vi "PeriodicFilter-Check Key.vi"(7 "seconds since 1Jan1904 2":timestamp, 10 "key":string, 11 "data in":T1 {"LastCheckT" format="%<%.3X>T"}) -> (0 "index":i32, 3 "data out":T1 {"LastCheckT" format="%<%.3X>T"})   [LabVIEW 2017, in "Communicable State Machine.lvlib"]
uses:
  Communicable State Machine.lvlib
  Periodic String Filter Data.ctl
  Periodic String Filter Info.ctl
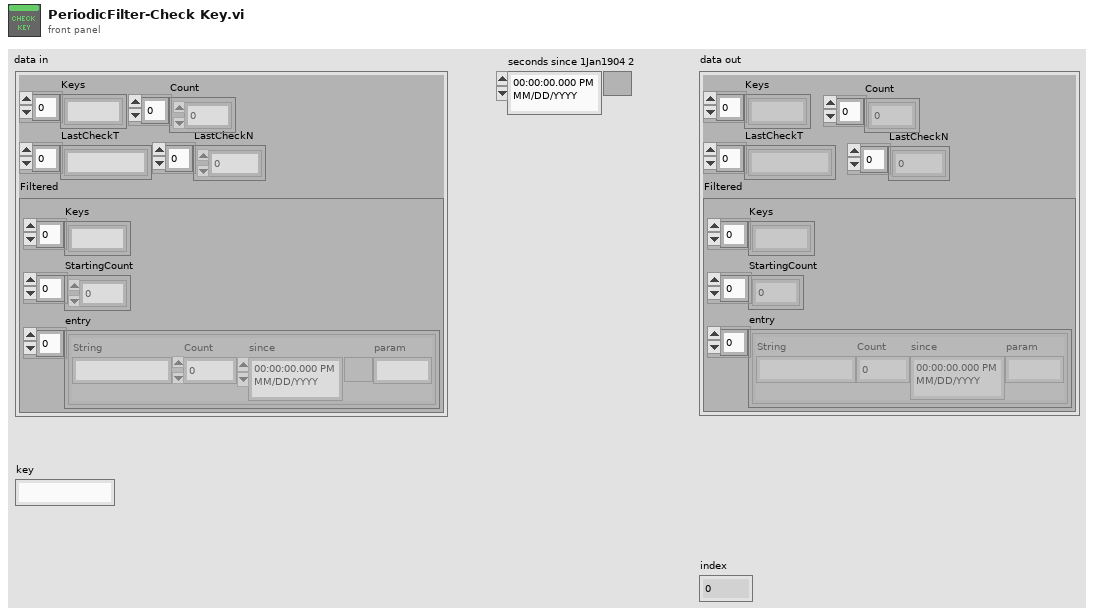
[diagram p1: front panel]
types:
  T1 = typedef "Communicable State Machine.lvlib/Periodic String Filter Data.ctl" = cluster{"Keys":string[], "Count":i64[], "LastCheckT":timestamp[], "LastCheckN":i64[], "Filtered":cluster{"Keys":string[], "StartingCount":i64[], "entry":T2[]}}
  T2 = typedef "Communicable State Machine.lvlib/Periodic String Filter Info.ctl" = cluster{"String":string, "Count":i64, "since":timestamp, "param":string}
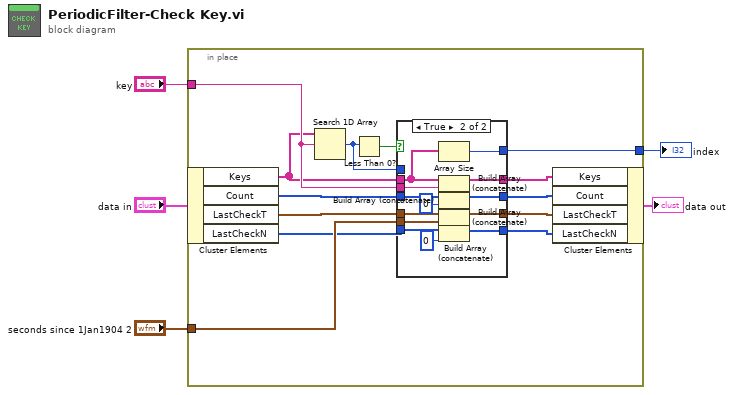
[diagram p0: block diagram]
diagram:
  n1 = in-place "In Place Element Structure" {
    in-place-border: "key" -> [w10]
    in-place-border: "seconds since 1Jan1904 2" -> [w13]
    in-place-border: [w6] -> w2
    n2 = in-place-cluster #1("data in") -> ("Keys"=w9:string[], "Count"=w17:i64[], "LastCheckT"=w15:timestamp[], "LastCheckN"=w12:i64[])
    n3 = Search 1D Array(1D array=w9, element=w10) -> (index of element=w7:i32)  [unwired: 1 in]
    n4 = Less Than 0?(x=w7) -> (x < 0?=w8:bool)
    n5 = case shown="True" w8 {
      tunnel: w9 -> [w23 w34]
      tunnel: w10 -> [_ w36]
      tunnel: [w23 w35] -> w18
      tunnel: w7 -> [w22 _]
      tunnel: [w22 w33] -> w6
      tunnel: w17 -> [w21 w32]
      tunnel: [w21 w30] -> w16
      tunnel: w15 -> [w20 w29]
      tunnel: w13 -> [_ w28]
      tunnel: [w20 w27] -> w14
      tunnel: w12 -> [w19 w26]
      tunnel: [w19 w24] -> w11
      frame False {
      }
      frame True {
        n6 = Array Size(array=w34) -> (size(s)=w33:i32)
        n7 = Build Array (concatenate)(w34, w36) -> (w35:string[])
        n8 = Build Array (concatenate)(w32, i64 0 ("64bit integer")) -> (w30:i64[])
        n9 = Build Array (concatenate)(w29, w28) -> (w27:timestamp[])
        n10 = Build Array (concatenate)(w26, i64 0 ("64bit integer")) -> (w24:i64[])
      }
    }
    n11 = in-place-cluster #1("Keys"=w18, "Count"=w16, "LastCheckT"=w14, "LastCheckN"=w11) -> (→"data out":T1)
  }
  "index" <- w2
